vi "Sample Rate 4.vi"() -> ()   [LabVIEW 2013]
uses:
  <vilib>/measure/NI_MABase.lvlib
panel:
  in  "Enum":enum16{"Sample Rate=400", "Sample Rate=1000"}(ring)
  out "Waveform Graph":waveform(dbl)(graph)
  in  "stop":bool
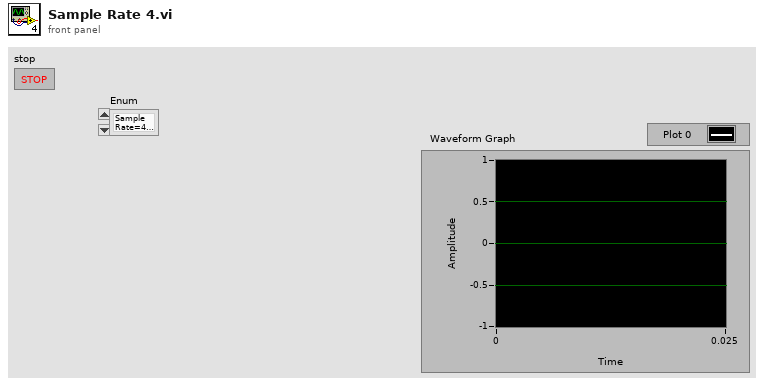
[diagram p1: front panel]
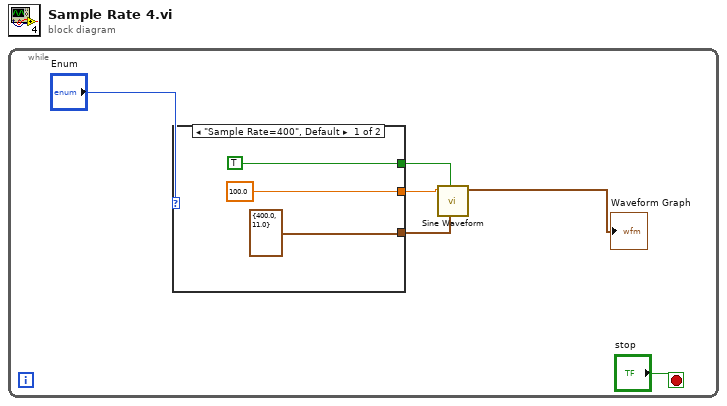
[diagram p0: block diagram]
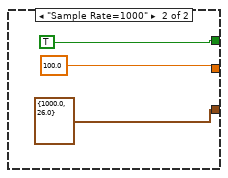
[diagram p2: hidden frame]
diagram:
  n1 = while {
    stop <- "stop" stop-if-true
    n2 = case shown="\"Sample Rate=400\", Default" "Enum" {
      tunnel: [cluster{"Fs":dbl, "#s":dbl} {"Fs"=400.0, "#s"=11.0} ("sampling info") cluster{"Fs":dbl, "#s":dbl} {"Fs"=1000.0, "#s"=26.0} ("sampling info")] -> w4
      tunnel: [100.0 100.0] -> w3
      tunnel: [TRUE TRUE] -> w2
      frame "Sample Rate=400", Default {
      }
      frame "Sample Rate=1000" {
      }
    }
    n3 = call <vilib>:"Sine Waveform.vi"("sampling info"=w4, "reset signal"=w2, "frequency"=w3) -> ("signal out"=→"Waveform Graph":waveform(dbl))  [unwired: 7 in, 1 out]
  }
